vi "FormatCoverLink.vi"(11 "Cover Link":string) -> (3 "result string":string)   [LabVIEW 2022 SP3]
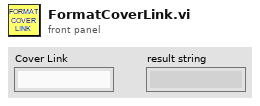
[diagram p1: front panel]
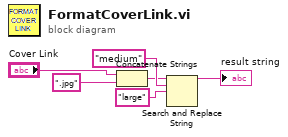
[diagram p0: block diagram]
diagram:
  n1 = Concatenate Strings("Cover Link", ".jpg" ("String")) -> (w1:string)
  n2 = Search and Replace String(input string=w1, search string="medium", replace string="large" ("replace string (\"\")")) -> (result string=→"result string":string)  [unwired: 5 in, 3 out]
